vi "encoderConsumer.vi"(8 "error in (no error)":errorcluster) -> (0 "error out":errorcluster)   [LabVIEW 2017, in "externalAquisition.lvlib"]
doc: "This VI is the Encoder consumer, which converts the raw string received via serial into the encoder counts.\n\nThe encoder counts are written to the 'All data' FGV."
uses:
  externalAquisition.lvlib
  internalQueue/TypeDefs/QueueCommands.ctl
  ErrorMonitor/ErrorMonitor.lvlib
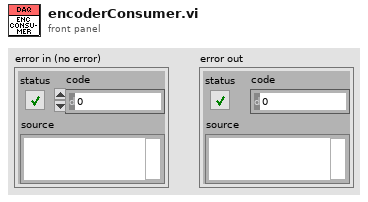
[diagram p1: front panel]
types:
  T1 = typedef "externalAquisition.lvlib/QueueCommands.ctl" = enum16{"obtain", "enqueue", "dequeue", "release"}
  T2 = typedef "dataOut.ctl" = cluster{"X0pos":dbl, "Y0pos":dbl, "Z0pos":dbl, "Fx":dbl, "Fy":dbl, "Fz":dbl, "Encoder1":i32, "Encoder2":i32, "Pot1":dbl, "Pot2":dbl, "Theta0":dbl, "Theta1":dbl, "X1pos":dbl, "Y1pos":dbl, "Z1pos":dbl, "X2pos":dbl, "Y2pos":dbl, "Z2pos":dbl, "ErrorOccurred":bool}
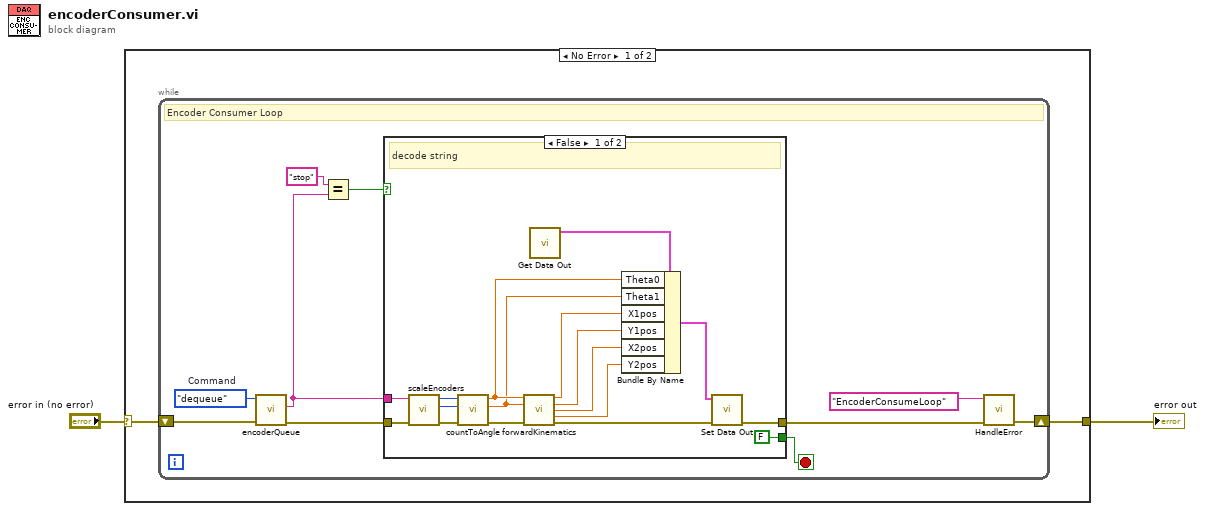
[diagram p0: block diagram]
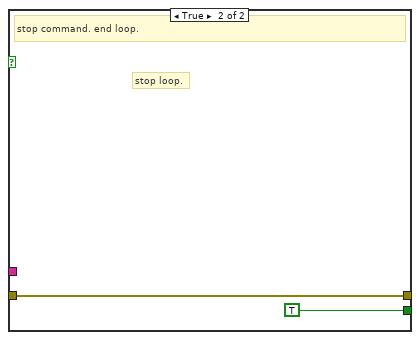
[diagram p2: hidden frame]
diagram:
  n1 = case shown="No Error" "error in (no error)" {
    selector: "error in (no error)" -> [w3 w34]
    tunnel: [w4 w34] -> w2
    frame No Error {
      n2 = while {
        shift-right: [w6] -> w4
        shift-left: w3 -> [w14]
        stop <- w9 stop-if-true
        w13 = QueueCommands."dequeue"  # Command
        # "Encoder Consumer Loop"
        n3 = call "encoderQueue.vi"("error in (no error)"=w14, "Command"=w13) -> ("error out"=w10:errorcluster, "encoderString"=w5:string)  [unwired: 8 in]
        n4 = Equal?(x="stop", y=w5) -> (x = y?=w11:bool)
        n5 = case shown="False" w11 {
          tunnel: w10 -> [w29 w33]
          tunnel: [w30 w33] -> w7
          tunnel: [FALSE TRUE] -> w9
          tunnel: w5 -> [w28 _]
          frame False {
            # "decode string"
            n6 = call "scaleEncoders.vi"("error in (no error)"=w29, "String"=w28) -> ("error out"=w25:errorcluster, "Encoder1"=w26:u32, "Encoder0"=w27:u32)  [unwired: 7 in]
            n7 = call "countToAngle.vi"("error in (no error)"=w25, "Encoder 1 Count"=w26, "Encoder 0 Count"=w27) -> ("error out"=w23:errorcluster, "Enc 1 angle (rad)"=w20:dbl, "Enc 0 angle (rad)"=w21:dbl)  [unwired: 6 in]
            n8 = call "forwardKinematics.vi"("Theta 0"=w21, "Theta 1"=w20, "error in (no error)"=w23) -> ("Link1X"=w19:dbl, "Link1Y"=w18:dbl, "Link2X"=w17:dbl, "Link2Y"=w16:dbl, "error out"=w22:errorcluster)  [unwired: 8 in]
            n9 = call "Get Data Out.vi"() -> ("DataOut"=w15:T2)  [unwired: 10 in, 1 out]
            n10 = Bundle By Name(cluster=w15, "Theta0"=w21, "Theta1"=w20, "X1pos"=w19, "Y1pos"=w18, "X2pos"=w17, "Y2pos"=w16) -> (w24:T2)
            n11 = call "Set Data Out.vi"("error in (no error)"=w22, "DataOut"=w24) -> ("error out"=w30:errorcluster)  [unwired: 9 in]
          }
          frame True {
            # "stop loop."
            # "stop command. end loop."
          }
        }
        n12 = call "HandleError.vi"("error in (no error)"=w7, "Source"="EncoderConsumeLoop") -> ("error out"=w6:errorcluster)  [unwired: 9 in]
      }
    }
    frame Error {
    }
  }
  "error out" <- w2
